vi "PC_Pub_imgFile initProperty.vi"(8 "error in (no error)":errorcluster, 11 "imgFile in":refnum<class "PC_Pub_imgFile.lvclass">) -> (0 "error out":errorcluster, 3 "imgFile out":refnum<class "PC_Pub_imgFile.lvclass">)   [LabVIEW 2018, in "PC_Pub_imgFile.lvclass"]
uses:
  PC_Pub_imgFile.lvclass
  <vilib>/Utility/miscctls.llb/LVRowAndColumnTypeDef.ctl
  PC_Pub_imgFile.lvclass/PC_Pub_imgFile.ctl
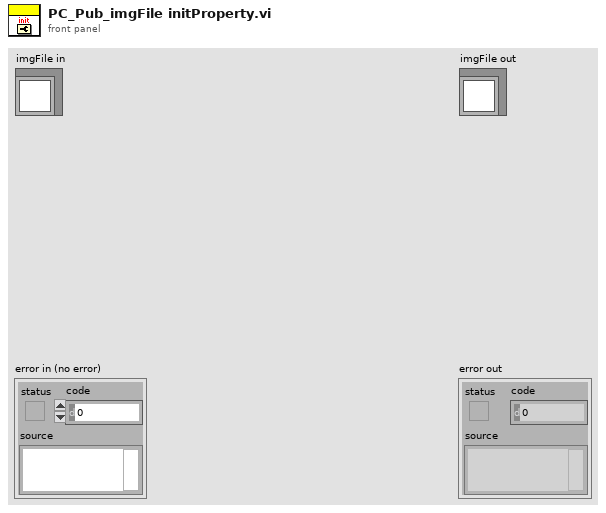
[diagram p1: front panel]
types:
  T1 = typedef "LVRowAndColumnTypeDef.ctl" = cluster{"Row":i32, "Column":i32}
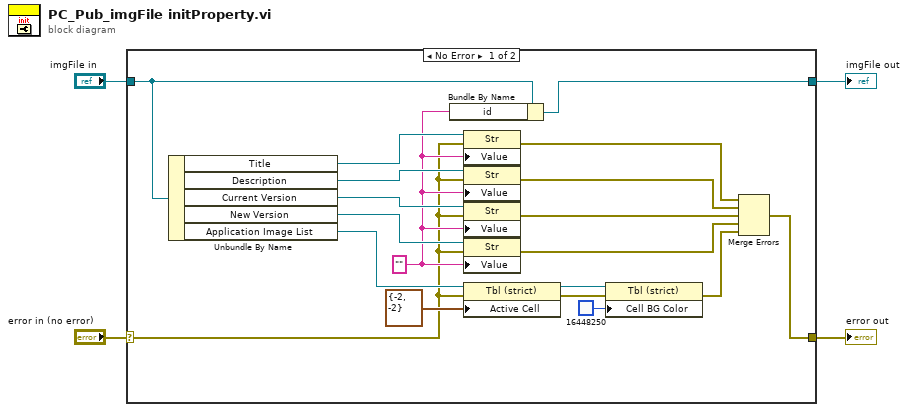
[diagram p0: block diagram]
diagram:
  n1 = case shown="No Error" "error in (no error)" {
    selector: "error in (no error)" -> [w5 w25]
    tunnel: [w12 w25] -> w3
    tunnel: [w17 w24] -> w1
    tunnel: "imgFile in" -> [w19 w24]
    frame No Error {
      w18 = "" ("Value")
      n2 = Unbundle By Name(w19) -> ("Title"=w23:refnum<vi>, "Description"=w22:refnum<vi>, "Current Version"=w21:refnum<vi>, "New Version"=w20:refnum<vi>, "Application Image List"=w7:refnum<vi>)
      n3 = Bundle By Name(cluster=w19, "id"=w18) -> (w17:refnum<class "PC_Pub_imgFile.lvclass">)
      n4 = property class="Str"(reference=w23, error in=w5, "Value"=w18) -> (error out=w16:errorcluster)  [unwired: 1 out]
      n5 = property class="Str"(reference=w22, error in=w5, "Value"=w18) -> (error out=w15:errorcluster)  [unwired: 1 out]
      n6 = property class="Str"(reference=w21, error in=w5, "Value"=w18) -> (error out=w14:errorcluster)  [unwired: 1 out]
      n7 = property class="Str"(reference=w20, error in=w5, "Value"=w18) -> (error out=w13:errorcluster)  [unwired: 1 out]
      n8 = property class="Tbl (strict)"(reference=w7, error in=w5, "Active Cell"=T1 {"Row"=-2, "Column"=-2} ("Active Cell:Active Cell")) -> (reference out=w10:refnum<vi>, error out=w9:errorcluster)
      n9 = property class="Tbl (strict)"(reference=w10, error in=w9, "Cell BG Color"=u32 16448250) -> (error out=w6:errorcluster)  [unwired: 1 out]
      n10 = Merge Errors(w16, w15, w14, w13, w6) -> (w12:errorcluster)
    }
    frame Error {
    }
  }
  "error out" <- w3
  "imgFile out" <- w1
